vi "GetItemInfo.vi"() -> (1 "ring info":refnum<class "RingItem.lvclass">[](array[class]), 3 "item info array":T1(array[cluster]))   [LabVIEW 2009, in "NavScreen.lvlib"]
uses:
  NavScreen.lvlib
  Classes/ClickableText/ClickableText.lvclass
  Classes/RingItem/RingItem.lvclass
panel:
  out "Debugging display - ring items - enable code on diagram to view":string[](array[string])
  out "Debugging display - enable code on diagram to view":cluster{string[]}[][](array[cluster])
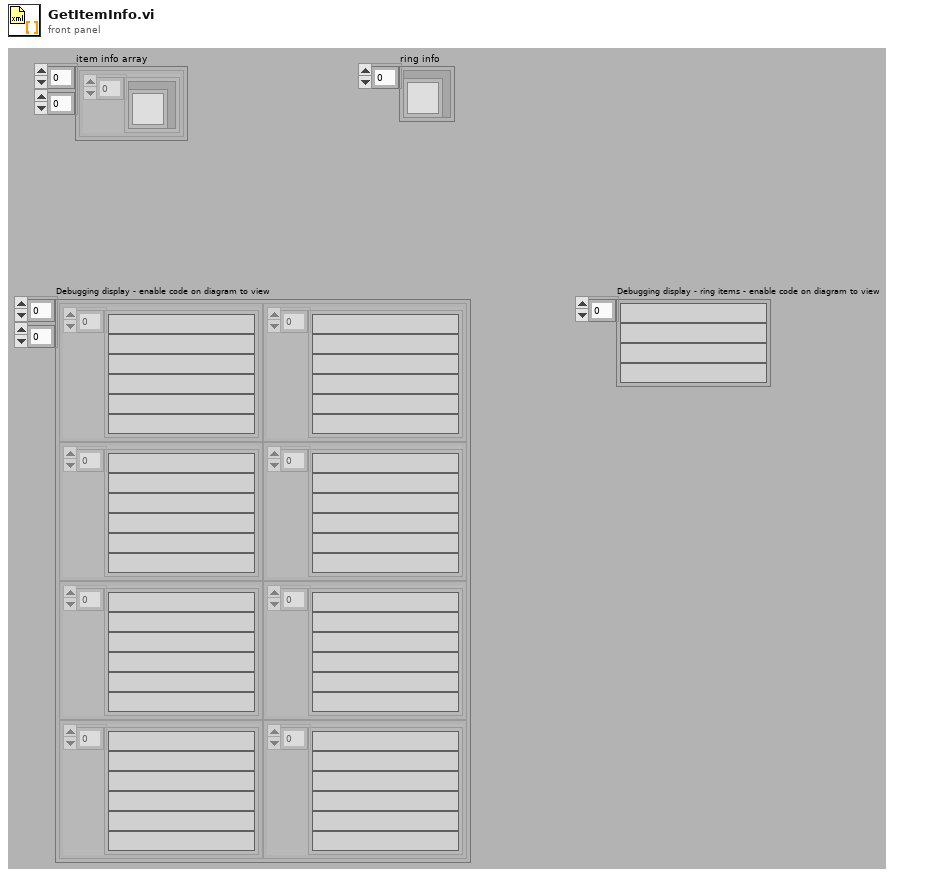
[diagram p1: front panel]
types:
  T1 = cluster{refnum<class "ClickableText.lvclass">[]}[][]
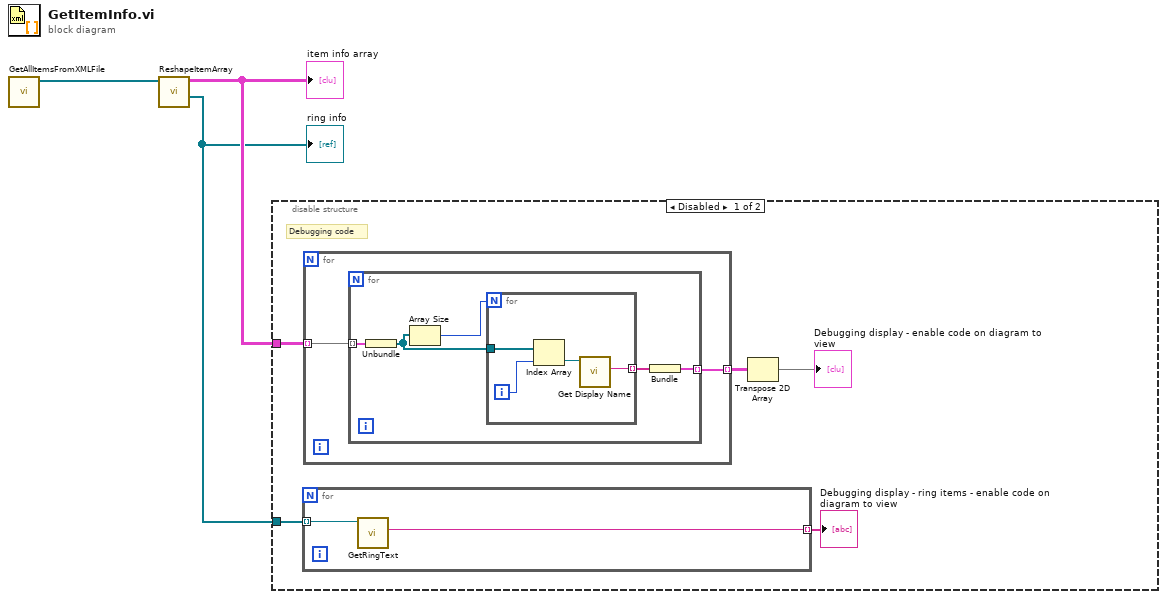
[diagram p0: block diagram]
diagram:
  n1 = call "GetAllItemsFromXMLFile.vi"() -> ("Array"=w1:refnum<class "Link.lvclass">[])  [unwired: 11 in]
  n2 = call "ReshapeItemArray.vi"("Array"=w1) -> ("ring info"=w2:refnum<class "RingItem.lvclass">[], "item info array"=w3:T1)  [unwired: 9 in]
  "item info array" <- w3
  "ring info" <- w2
  n3 = disable-structure shown="Disabled" {
    disable-tunnel: w3 -> [w8 _]
    disable-tunnel: w2 -> [w7 _]
    frame #0 {
      # "Debugging code"
      n4 = for {
        tunnel: w7 -> [w10] mode=indexing
        tunnel: [w9] -> w6 mode=indexing
        n5 = call "GetRingText.vi"("RingItem in"=w10) -> ("ring text"=w9:string)  [unwired: 8 in, 2 out]
      }
      "Debugging display - ring items - enable code on diagram to view" <- w6
      n6 = for {
        tunnel: w8 -> [w12] mode=indexing
        tunnel: [w11] -> w5 mode=indexing
        n7 = for {
          tunnel: w12 -> [w17] mode=indexing
          tunnel: [w13] -> w11 mode=indexing
          n8 = Unbundle(w17) -> (w15:refnum<class "ClickableText.lvclass">[])
          n9 = Array Size(array=w15) -> (size(s)=w16:i32)
          n10 = for {
            N: w16 -> [_]
            tunnel: w15 -> [w21]
            tunnel: [w18] -> w14 mode=indexing
            i -> [w20]
            n11 = Index Array(array=w21, index=w20) -> (element=w19:refnum<class "ClickableText.lvclass">)
            n12 = call-dynamic "Get Display Name.vi"("ClickableText in"=w19) -> ("localized name"=w18:string)  [unwired: 8 in, 2 out]
          }
          n13 = Bundle(w14) -> (w13:cluster{string[]})  [unwired: 1 in]
        }
      }
      n14 = Transpose 2D Array(2D array=w5) -> (transposed array=→"Debugging display - enable code on diagram to view":cluster{string[]}[][])
    }
    frame #1 {
    }
  }
